vi "myRIO_BRig_FPGA_lick.vi"(8 "I_stateDetector_new":bool, 10 "counter":u32, 11 "I_stateDetector_prev":bool) -> (0 "output_I_lick":bool, 2 "output_counter":u32, 3 "output_I_stateDetector_prev":bool)   [LabVIEW 2014]
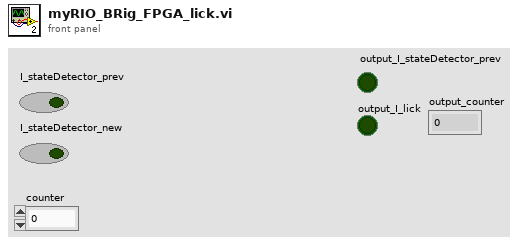
[diagram p1: front panel]
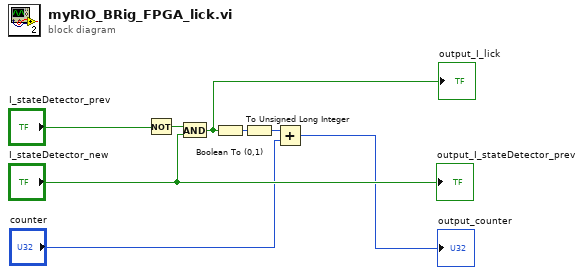
[diagram p0: block diagram]
diagram:
  n1 = Not(x="I_stateDetector_prev") -> (.not. x?=w5:bool)
  n2 = And(x=w5, y="I_stateDetector_new") -> (x .and. y?=w7:bool)
  "output_I_lick" <- w7
  n3 = Boolean To (0,1)(Boolean=w7) -> (0, 1=w8:i16)
  n4 = To Unsigned Long Integer(number=w8) -> (unsigned 32bit integer=w6:u32)
  n5 = Add(x=w6, y="counter") -> (x+y=→"output_counter":u32)
  "output_I_stateDetector_prev" <- "I_stateDetector_new"
